vi "read_new_data.vi"(8 "Error In":errorcluster, 9 "connected?":bool, 10 "VISA in":refnum<visa-resource-name>, 11 "Data Cluster In":T1) -> (0 "Error Out":errorcluster, 2 "VISA out":refnum<visa-resource-name>, 3 "Data Cluster Out":T1)   [LabVIEW 2019]
uses:
  data_cluster_typedef.ctl
panel:
  out "Serial Settings:Number of Bytes at Serial Port":u32
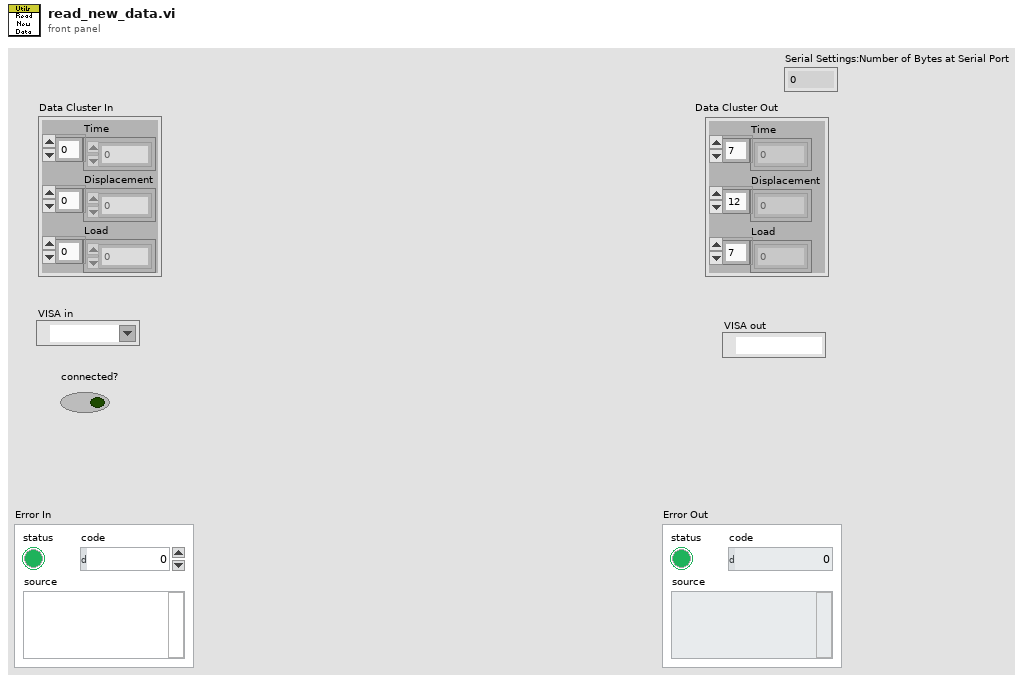
[diagram p1: front panel]
types:
  T1 = typedef "data_cluster_typedef.ctl" = cluster{"Time":dbl[], "Displacement":dbl[], "Load":dbl[]}
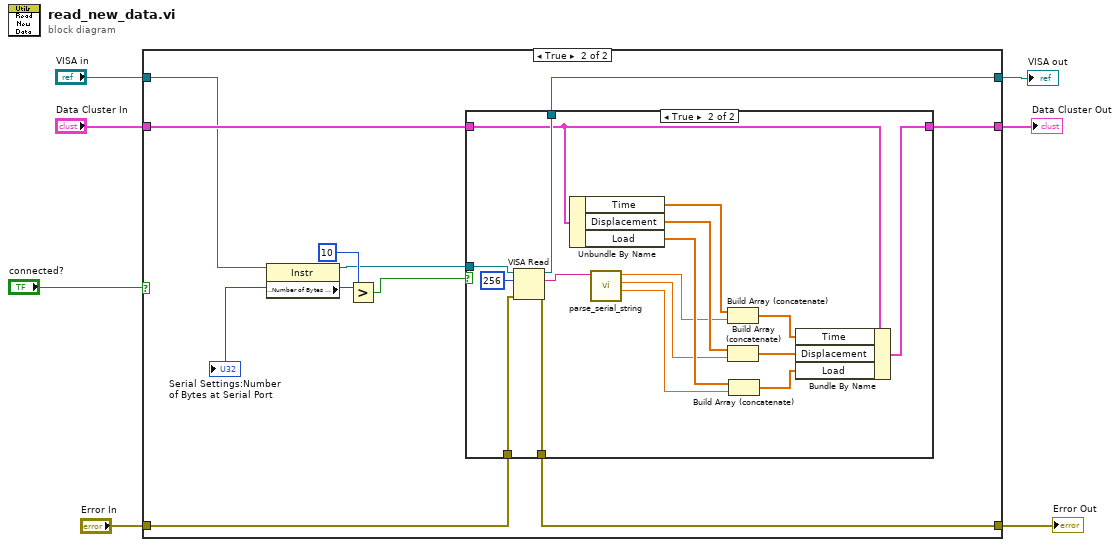
[diagram p0: block diagram]
diagram:
  n1 = case shown="True" "connected?" {
    tunnel: [w10 w20] -> w6
    tunnel: "VISA in" -> [w10 w15]
    tunnel: "Data Cluster In" -> [w9 w18]
    tunnel: [w9 w17] -> w3
    tunnel: "Error In" -> [w8 w19]
    tunnel: [w8 w16] -> w1
    frame False {
      # "Not connected - so just keep passing everything\nthough to keep the graphs, etc populated."
    }
    frame True {
      n2 = property class="Instr"(reference=w15) -> (reference out=w11:refnum<visa-resource-name>, "Serial Settings:Number of Bytes at Serial Port"=w14:u32)  [unwired: 1 in, 1 out]
      "Serial Settings:Number of Bytes at Serial Port" <- w14
      n3 = Greater?(x=w14, y=u32 10) -> (0:w12:bool)
      n4 = case shown="True" w12 {
        tunnel: [w23 w40] -> w20
        tunnel: w19 -> [w22 w39]
        tunnel: w18 -> [w21 w35]
        tunnel: [w21 w34] -> w17
        tunnel: [w22 w33] -> w16
        tunnel: w11 -> [w23 w31]
        frame False {
        }
        frame True {
          n5 = VISA Read(VISA resource name=w31, byte count=u32 256, error in (no error)=w39) -> (VISA resource name out=w40:refnum<visa-resource-name>, read buffer=w27:string, error out=w33:errorcluster)  [unwired: 1 out]
          n6 = Unbundle By Name(w35) -> ("Time"=w38:dbl[], "Displacement"=w37:dbl[], "Load"=w36:dbl[])
          n7 = call "parse_serial_string.vi"("Input String"=w27) -> ("Load"=w24:dbl, "Displacement"=w25:dbl, "Time"=w26:dbl)  [unwired: 7 in, 1 out]
          n8 = Build Array (concatenate)(w38, w26) -> (w30:dbl[])
          n9 = Build Array (concatenate)(w37, w25) -> (w29:dbl[])
          n10 = Build Array (concatenate)(w36, w24) -> (w28:dbl[])
          n11 = Bundle By Name(cluster=w35, "Time"=w30, "Displacement"=w29, "Load"=w28) -> (w34:T1)
        }
      }
    }
  }
  "Error Out" <- w1
  "Data Cluster Out" <- w3
  "VISA out" <- w6
